vi "image correction.vi"(1 "Image":T1) -> (0 "ref points":T2)   [LabVIEW 2014]
uses:
  <vilib>/vision/Image Controls.llb/IMAQ Image.ctl
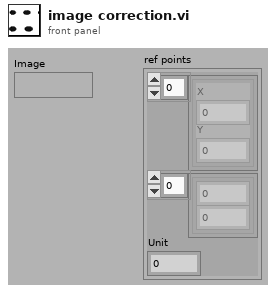
[diagram p1: front panel]
types:
  T1 = typedef "IMAQ Image.ctl" = refnum<image>
  T2 = cluster{cluster{"X":sgl, "Y":sgl}[], cluster{i32, i32}[], "Unit":u32}
  T3 = typedef "IMAQ Point" = cluster{"X":sgl, "Y":sgl}
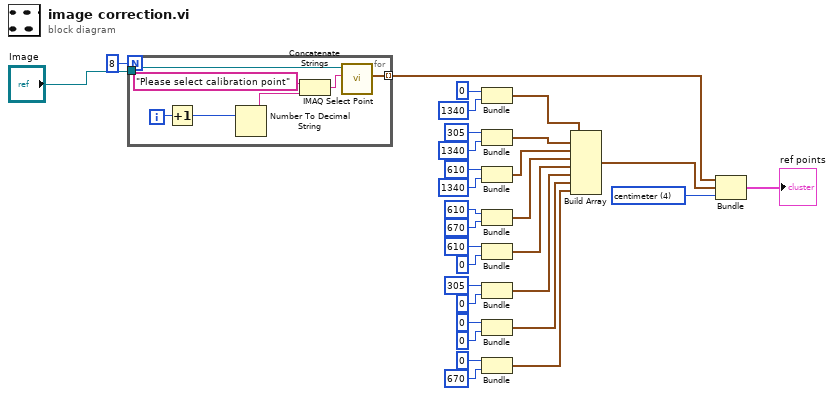
[diagram p0: block diagram]
diagram:
  w26 = u32 4 items=["Undefined", "Angstrom", "micrometer", "millimeter", "centimeter", "meter", "kilometer", "microinch", "inch", "feet", "nautic miles", "standard miles", "steps"] ("Unit")
  n1 = for {
    N: 8 -> [_]
    tunnel: "Image" -> [w37]
    tunnel: [w31] -> w3 mode=indexing
    i -> [w36]
    n2 = Increment(x=w36) -> (x+1=w33:i32)
    n3 = Number To Decimal String(number=w33) -> (decimal integer string=w32:string)  [unwired: 1 in]
    n4 = Concatenate Strings("Please select calibration point" ("string"), w32) -> (w34:string)
    n5 = call "IMAQ Select Point"("Prompt"=w34, "Image In"=w37) -> ("Point"=w31:T3)  [unwired: 6 in, 3 out]
  }
  n6 = Bundle(0, 1340) -> (w28:cluster{i32, i32})  [unwired: 1 in]
  n7 = Bundle(305, 1340) -> (w10:cluster{i32, i32})  [unwired: 1 in]
  n8 = Bundle(610, 1340) -> (w9:cluster{i32, i32})  [unwired: 1 in]
  n9 = Bundle(610, 670) -> (w8:cluster{i32, i32})  [unwired: 1 in]
  n10 = Bundle(610, 0) -> (w7:cluster{i32, i32})  [unwired: 1 in]
  n11 = Bundle(305, 0) -> (w6:cluster{i32, i32})  [unwired: 1 in]
  n12 = Bundle(0, 0) -> (w5:cluster{i32, i32})  [unwired: 1 in]
  n13 = Bundle(0, 670) -> (w4:cluster{i32, i32})  [unwired: 1 in]
  n14 = Build Array(w28, w10, w9, w8, w7, w6, w5, w4) -> (w27:cluster{i32, i32}[])
  n15 = Bundle(w3, w27, "Unit"=w26) -> (→"ref points":cluster{T3[], cluster{i32, i32}[], "Unit":u32})  [unwired: 1 in]
